vi "write device information.vi"(8 "error in":errorcluster, 10 "device information":T1, 11 "Controller in":refnum<class "Controller.lvclass">) -> (0 "error out":errorcluster, 3 "Controller out":refnum<class "Controller.lvclass">)   [LabVIEW 2016, in "SMI.lvlib" / "Controller.lvclass"]
uses:
  Controller.lvclass
  device information.ctl
  Controller.lvclass/Controller.ctl
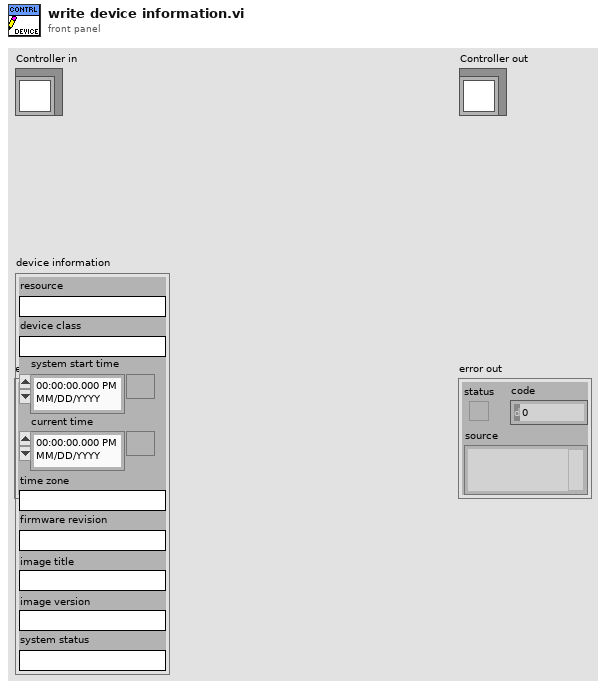
[diagram p1: front panel]
types:
  T1 = typedef "SMI.lvlib/Controller.lvclass/device information.ctl" = cluster{"resource":string, "device class":string, "system start time":timestamp, "current time":timestamp, "time zone":string, "firmware revision":string, "image title":string, "image version":string, "system status":string}
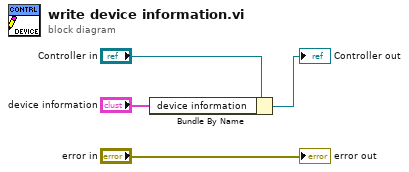
[diagram p0: block diagram]
diagram:
  n1 = Bundle By Name(cluster="Controller in", "device information"="device information") -> (→"Controller out":refnum<class "Controller.lvclass">)
  "error out" <- "error in"
